vi "Toggle.vi"(1 "Initial State":bool, 2 "Trigger":bool) -> (0 "New State":bool)   [LabVIEW 2019]
doc: "When the Trigger input is set to TRUE (rising edge), the output New State toggles its Boolean value. The Initial Value of the state can be configured."
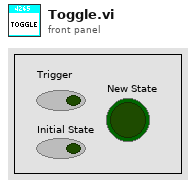
[diagram p1: front panel]
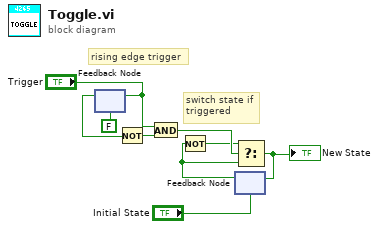
[diagram p0: block diagram]
diagram:
  # "rising edge trigger"
  # "switch state if\ntriggered"
  n1 = feedback-in #1("Trigger") -> ()
  n2 = feedback #1(FALSE ("Button")) -> (w5:bool)
  n3 = Not(x=w5) -> (.not. x?=w7:bool)
  n4 = And(x="Trigger", y=w7) -> (x .and. y?=w9:bool)
  n5 = feedback #2("Initial State") -> (w3:bool)
  n6 = Not(x=w3) -> (.not. x?=w8:bool)
  n7 = Select(t=w8, s=w9, f=w3) -> (s? t:f=w4:bool)
  "New State" <- w4
  n8 = feedback-in #2(w4) -> ()
